vi "Drive_Constants.vi"() -> (19 "Camera Offset":dbl=0.5, 20 "Position accuracy (m)":dbl=0.05, 21 "Speed step (m/s)":dbl=0.005, 22 "Wheels interval (m)":dbl=0.6, 23 "Speed convert constant":dbl=0.6, 24 "Position control loop period (ms)":i64, 25 "Turning correction constant":dbl=0.05, 26 "Maximum angle step":dbl=2.5, 27 "Angle accuracy":dbl=0.03)   [LabVIEW 2009, in "Drive.lvlib" / "Drive_Utils.lvlib"]
doc: "This VI contains the parameters used in robot driving"
uses:
  Drive_Utils.lvlib
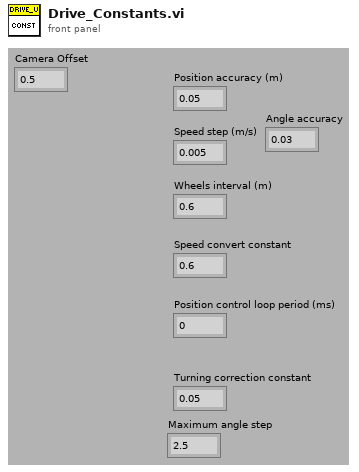
[diagram p1: front panel]
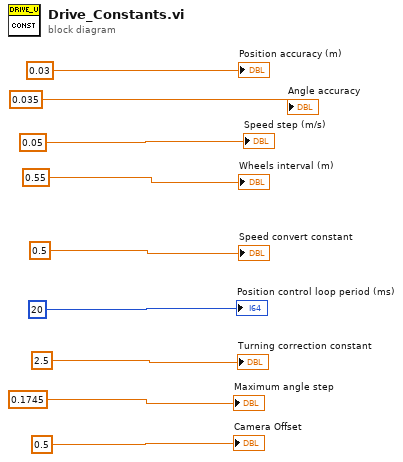
[diagram p0: block diagram]
diagram:
  "Position accuracy (m)" <- 0.03 ("Position accuracy")
  "Speed step (m/s)" <- 0.05 ("Position accuracy")
  "Wheels interval (m)" <- 0.55 ("Wheels interval")
  "Speed convert constant" <- 0.5 ("Speed convert constant")
  "Position control loop period (ms)" <- i64 20 ("Position control loop period")
  "Turning correction constant" <- 2.5 ("Turning correction constance")
  "Maximum angle step" <- 0.1745 ("Turning correction constance")
  "Angle accuracy" <- 0.035 ("Position accuracy")
  "Camera Offset" <- 0.5 ("Turning correction constance")
